vi "CloseOnSDLQuit-Set.vi"(8 "error in (no error)":errorcluster, 10 "Close On SDL Quit?":bool, 11 "Engine in":refnum<class "Engine.lvclass">) -> (0 "error out":errorcluster, 3 "Engine out":refnum<class "Engine.lvclass">)   [LabVIEW 2024, in "GLF.lvlib" / "Engine.lvclass"]
uses:
  Engine.lvclass
  Engine.lvclass/Engine.ctl
  DataMember--enum.ctl
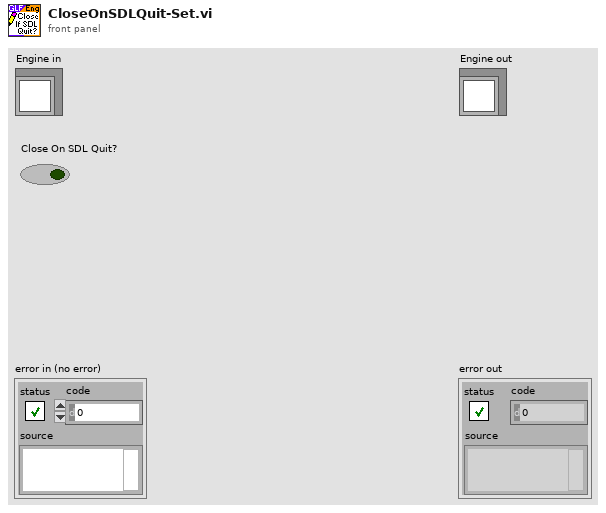
[diagram p1: front panel]
types:
  T1 = typedef "GLF.lvlib/Engine.lvclass/DataMember--enum.ctl" = enum16{"Close On SDL Quit?"}
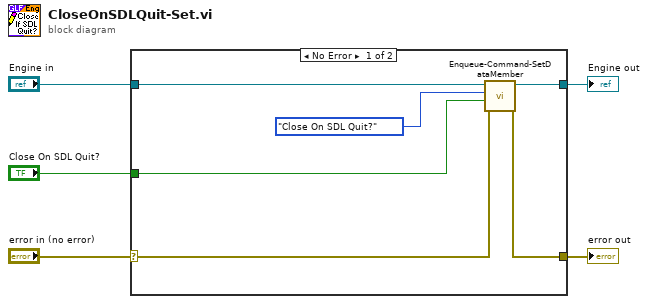
[diagram p0: block diagram]
diagram:
  n1 = case shown="No Error" "error in (no error)" {
    selector: "error in (no error)" -> [w9 w12]
    tunnel: [w8 w12] -> w4
    tunnel: [w10 w13] -> w2
    tunnel: "Engine in" -> [w11 w13]
    tunnel: "Close On SDL Quit?" -> [w6 _]
    frame No Error {
      n2 = call "Enqueue-Command-SetDataMember.vi"("error in (no error)"=w9, "Data Member Value"=w6, "Data Member"=DataMember--enum."Close On SDL Quit?", "Engine in"=w11) -> ("error out"=w8:errorcluster, "Engine out"=w10:refnum<class "Engine.lvclass">)  [unwired: 5 in, 1 out]
    }
    frame Error {
    }
  }
  "error out" <- w4
  "Engine out" <- w2
